vi "Number To Match.vi"() -> ()   [LabVIEW 2021]
panel:
  in  "stop":bool
  out "Iteration Count":dbl
  in  "Number To Match":dbl
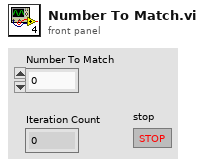
[diagram p1: front panel]
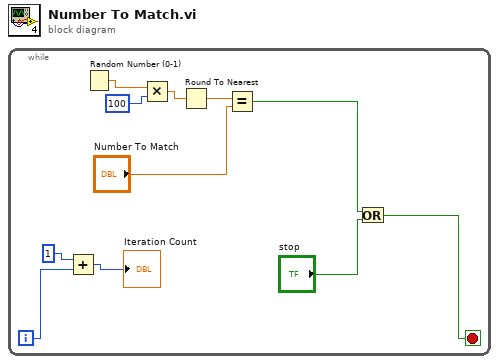
[diagram p0: block diagram]
diagram:
  n1 = while {
    i -> [w11]
    stop <- w1 stop-if-true
    n2 = Add(x=1, y=w11) -> (x+y=→"Iteration Count":i32)
    n3 = Random Number (0-1)() -> (number: 0 to 1=w7:dbl)
    n4 = Multiply(x=w7, y=100) -> (x*y=w5:dbl)
    n5 = Round To Nearest(number=w5) -> (nearest integer value=w4:dbl)
    n6 = Equal?(x=w4, y="Number To Match") -> (x = y?=w3:bool)
    n7 = Or(x=w3, y="stop") -> (x .or. y?=w1:bool)
  }
